vi "AB_RW_Project_Source_ExportedAssemblyVI.vi"(7 "action":T5, 8 "error in (no error)":errorcluster, 9 "index in":i32, 10 "dataSource in":T2, 11 "buildObject":T1) -> (0 "error out":errorcluster, 1 "index out":i32, 2 "dataSource out":T2, 3 "buildObject out":T1)   [LabVIEW 2020]
doc: "Reads and writes the data to the object property bag."
uses:
  <vilib>/AppBuilder/RW_Project/AB_RW_Project_PropBag_Action.ctl
  <vilib>/AppBuilder/RW_Project/AB_RW_Project_Source_ExportedAssemblyVI_Data.ctl
  <vilib>/AppBuilder/AB_InteropAssembly_DistVI_Proto_Info.ctl
  <vilib>/AppBuilder/IOStatus.ctl
  <resource>/Framework/Providers/API/ItemRef.ctl
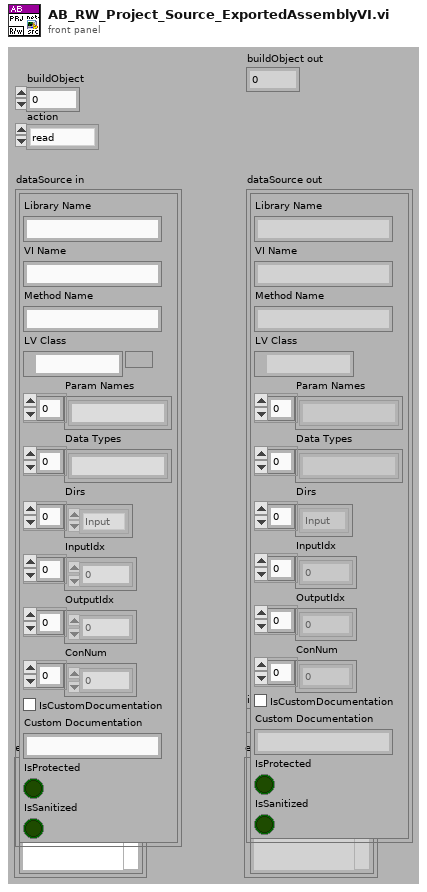
[diagram p1: front panel]
types:
  T1 = typedef "ItemRef.ctl" = u64
  T2 = typedef "AB_RW_Project_Source_ExportedAssemblyVI_Data.ctl" = cluster{"ExportAssemblyVIinfo":T3}
  T3 = typedef "AB_InteropAssembly_DistVI_Proto_Info.ctl" = cluster{"Library Name":string, "VI Name":string, "Method Name":string, "LV Class":path, "Param Names":string[], "Data Types":string[], "Dirs":T4[], "InputIdx":i32[], "OutputIdx":i32[], "ConNum":i8[], "IsCustomDocumentation":bool, "Custom Documentation":string, "IsProtected":bool, "IsSanitized":bool}
  T4 = typedef "IOStatus.ctl" = enum16{"Input", "Output", "Input/Output", "InputDeleted", "OutputDeleted", "IODeleted", "ErrorClusterIn", "ErrorClusterOut"}
  T5 = typedef "AB_RW_Project_PropBag_Action.ctl" = enum16{"read", "write", "clear", "readPrevious", "writePrevious", "clearPrevious"}
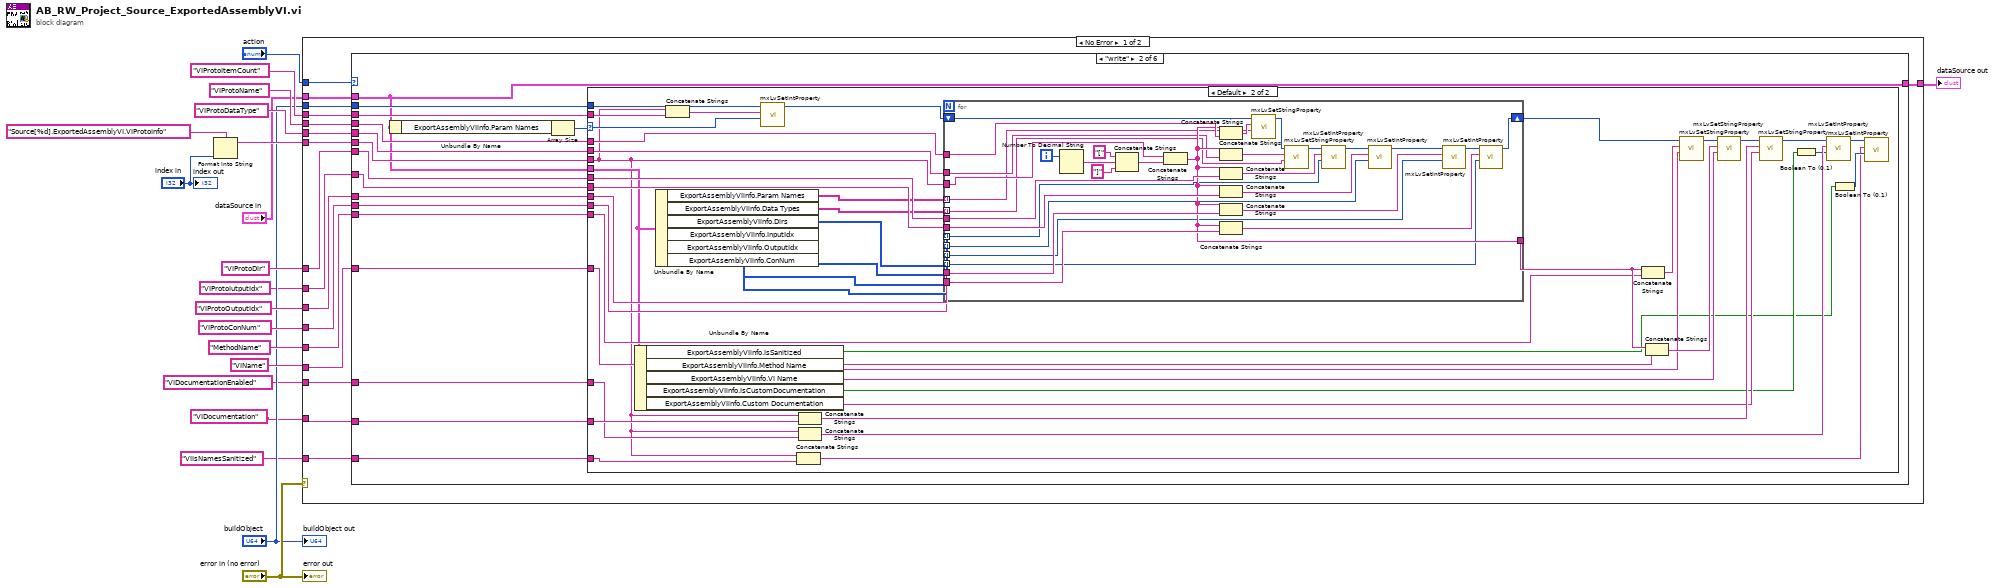
[diagram p0: block diagram]
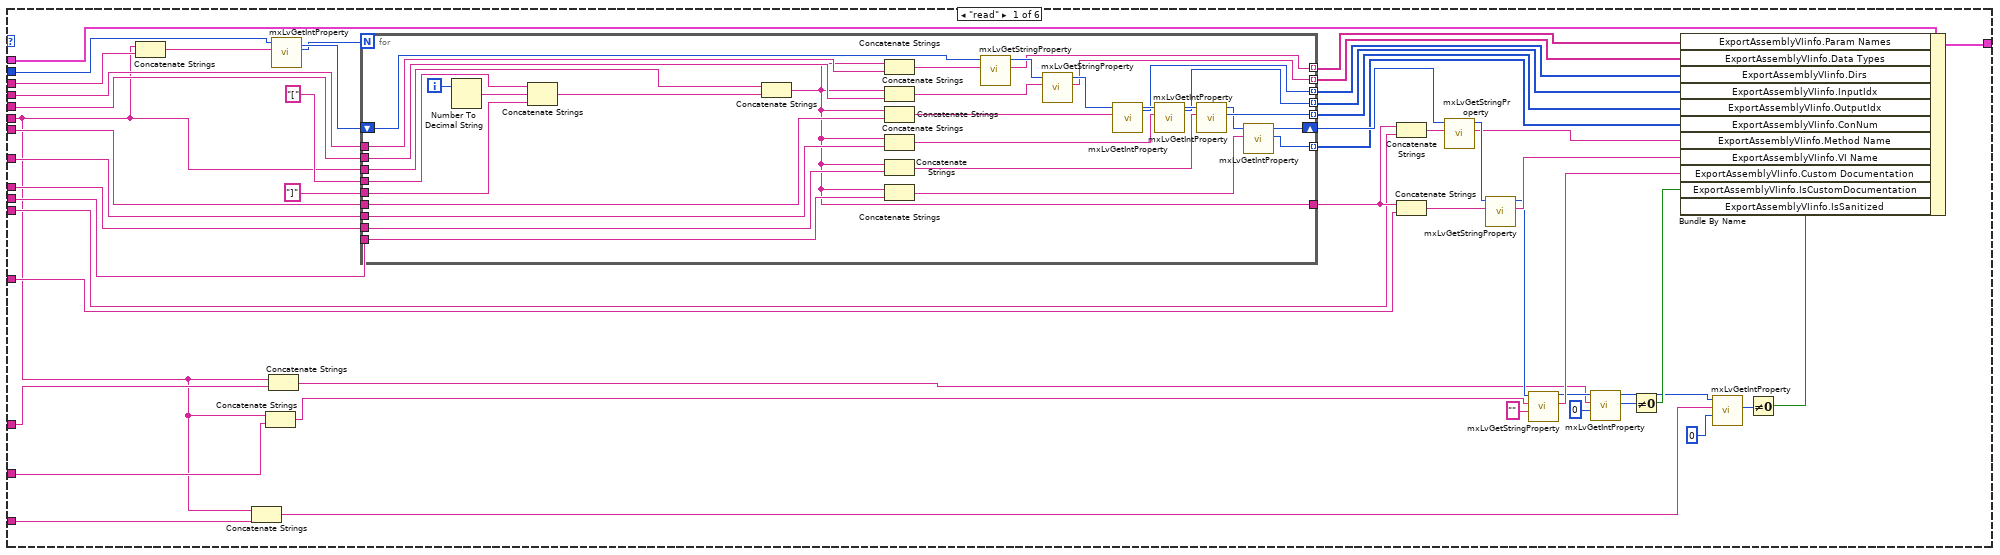
[diagram p2: hidden frame]
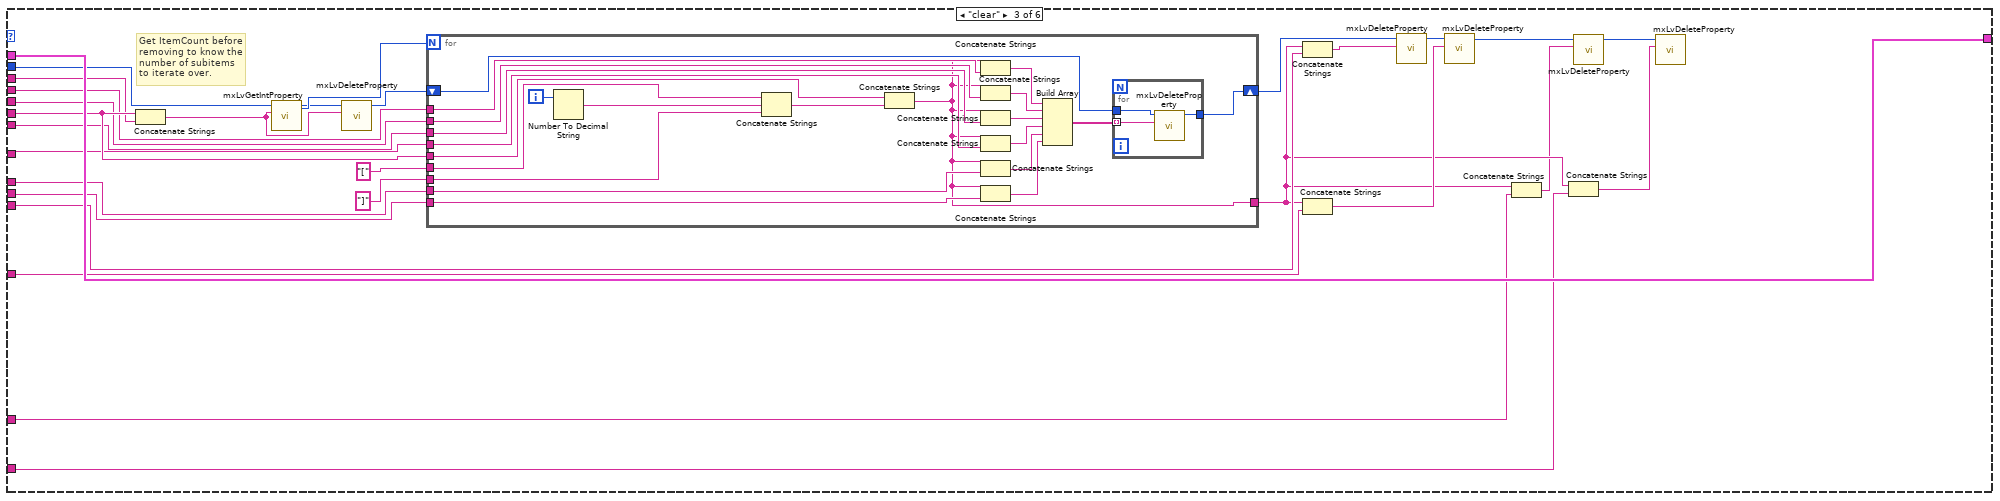
[diagram p4: hidden frame]
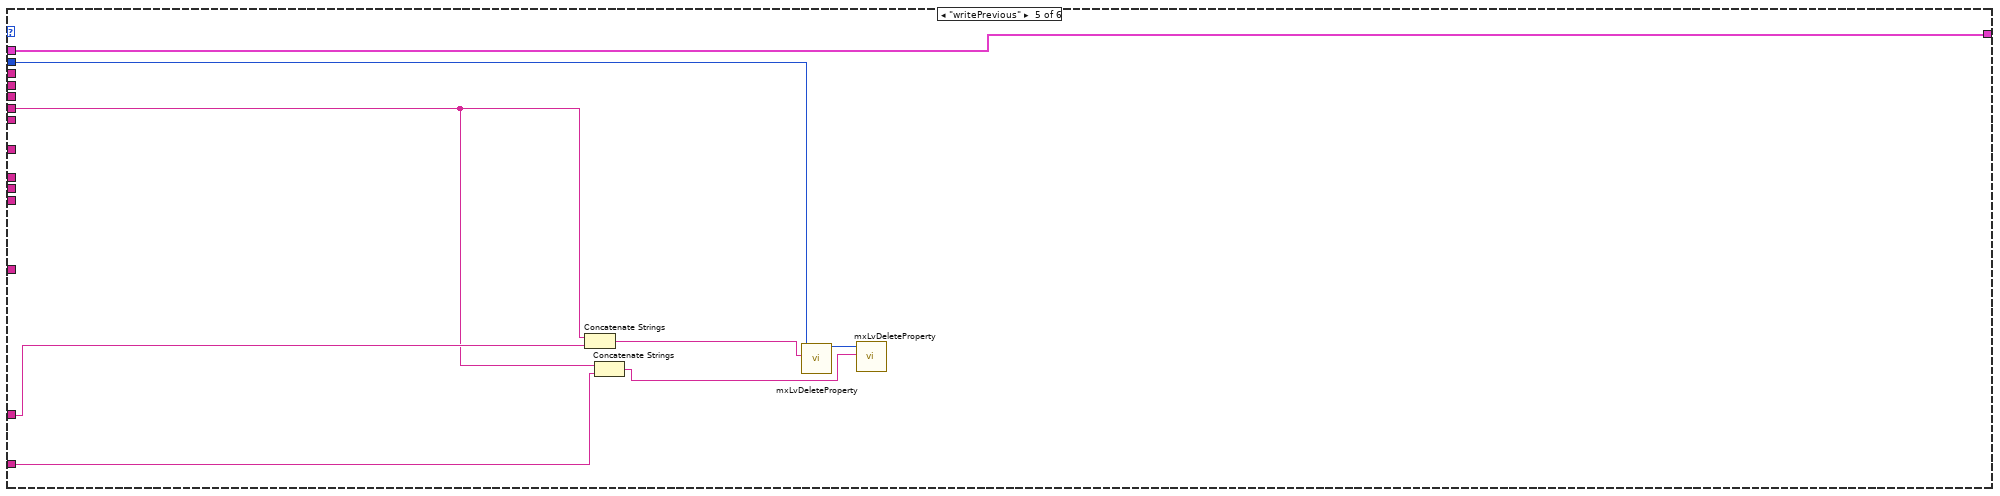
[diagram p6: hidden frame]
diagram:
  n1 = Format Into String(format string="Source[%d].ExportedAssemblyVI.VIProtoInfo", "index in") -> (resulting string=w18:string)  [unwired: 2 in, 1 out]
  n2 = case shown="No Error" "error in (no error)" {
    tunnel: "action" -> [w37 _]
    tunnel: "dataSource in" -> [w36 w273]
    tunnel: w18 -> [w35 _]
    tunnel: "buildObject" -> [w34 _]
    tunnel: [w33 w273] -> w6
    tunnel: "VIProtoItemCount" -> [w32 _]
    tunnel: "VIProtoName" ("string") -> [w31 _]
    tunnel: "VIProtoDataType" ("string") -> [w30 _]
    tunnel: "VIProtoDir" ("string") -> [w29 _]
    tunnel: "VIProtoOutputIdx" ("string") -> [w28 _]
    tunnel: "VIProtoConNum" ("string") -> [w27 _]
    tunnel: "MethodName" -> [w26 _]
    tunnel: "VIName" -> [w25 _]
    tunnel: "VIProtoIutputIdx" ("string") -> [w24 _]
    tunnel: "VIDocumentation" -> [w23 _]
    tunnel: "VIDocumentationEnabled" -> [w22 _]
    tunnel: "VIIsNamesSanitized" -> [w21 _]
    frame No Error {
      n3 = case shown="\"write\"" w37 {
        tunnel: w34 -> [w70 w132 w217 _ w267 _]
        tunnel: w36 -> [w57 w121 w237 w263 w271 w272]
        tunnel: w35 -> [w40 w133 w236 _ w266 _]
        tunnel: [w56 w121 w237 w263 w271 w272] -> w33
        tunnel: w32 -> [w78 w130 w235 _ _ _]
        tunnel: w31 -> [w77 w131 w224 _ _ _]
        tunnel: w30 -> [w76 w128 w223 _ _ _]
        tunnel: w29 -> [w75 w127 w222 _ _ _]
        tunnel: w28 -> [w74 w126 w221 _ _ _]
        tunnel: w27 -> [w73 w125 w220 _ _ _]
        tunnel: w26 -> [w72 w124 w218 _ _ _]
        tunnel: w25 -> [w71 w123 w219 _ _ _]
        tunnel: w24 -> [w69 w122 w216 _ _ _]
        tunnel: w23 -> [w55 w120 w210 _ w265 _]
        tunnel: w22 -> [w54 w119 w211 _ w270 _]
        tunnel: w21 -> [w39 w118 _ _ _ _]
        frame "read" {
          n4 = Concatenate Strings(w40, w78) -> (w84:string)
          n5 = Concatenate Strings(w40, w39) -> (w38:string)
          n6 = Concatenate Strings(w40, w55) -> (w53:string)
          n7 = Concatenate Strings(w40, w54) -> (w47:string)
          n8 = call <resource>:"mxLvGetIntProperty.vi"("Tag"=w84, "Item"=w70) -> ("Value"=w79:i32, "Item"=w83:T1)  [unwired: 1 in, 7 out]
          n9 = for {
            N: w79 -> [_]
            tunnel: "[" -> [w116]
            tunnel: "]" -> [w115]
            tunnel: w40 -> [w111]
            tunnel: [w100] -> w80
            shift-right: [w93] -> w68
            shift-left: w83 -> [w113]
            tunnel: w77 -> [w106]
            tunnel: w76 -> [w105]
            tunnel: w75 -> [w104]
            tunnel: w74 -> [w103]
            tunnel: w73 -> [w102]
            tunnel: w69 -> [w101]
            tunnel: [w92] -> w65 mode=indexing
            tunnel: [w91] -> w64 mode=indexing
            tunnel: [w90] -> w63 mode=indexing
            tunnel: [w89] -> w62 mode=indexing
            tunnel: [w88] -> w61 mode=indexing
            tunnel: [w87] -> w60 mode=indexing
            i -> [w114]
            n10 = Number To Decimal String(number=w114) -> (decimal integer string=w117:string)  [unwired: 1 out]
            n11 = Concatenate Strings(w116, w117, w115) -> (w110:string)
            n12 = Concatenate Strings(w111, w110) -> (w100:string)
            n13 = Concatenate Strings(w100, w106) -> (w112:string)
            n14 = Concatenate Strings(w100, w105) -> (w97:string)
            n15 = Concatenate Strings(w100, w104) -> (w109:string)
            n16 = Concatenate Strings(w100, w101) -> (w94:string)
            n17 = Concatenate Strings(w100, w103) -> (w108:string)
            n18 = Concatenate Strings(w100, w102) -> (w107:string)
            n19 = call <resource>:"mxLvGetStringProperty.vi"("Tag"=w112, "Item"=w113) -> ("Value"=w92:string, "Item"=w99:T1)  [unwired: 1 in, 7 out]
            n20 = call <resource>:"mxLvGetStringProperty.vi"("Tag"=w97, "Item"=w99) -> ("Value"=w91:string, "Item"=w98:T1)  [unwired: 1 in, 7 out]
            n21 = call <resource>:"mxLvGetIntProperty.vi"("Tag"=w109, "Item"=w98) -> ("Value"=w90:i32, "Item"=w95:T1)  [unwired: 1 in, 7 out]
            n22 = call <resource>:"mxLvGetIntProperty.vi"("Tag"=w94, "Item"=w95) -> ("Value"=w89:i32, "Item"=w96:T1)  [unwired: 1 in, 7 out]
            n23 = call <resource>:"mxLvGetIntProperty.vi"("Tag"=w108, "Item"=w96) -> ("Value"=w88:i32, "Item"=w86:T1)  [unwired: 1 in, 7 out]
            n24 = call <resource>:"mxLvGetIntProperty.vi"("Tag"=w107, "Item"=w86) -> ("Value"=w87:i32, "Item"=w93:T1)  [unwired: 1 in, 7 out]
          }
          n25 = Concatenate Strings(w80, w72) -> (w66:string)
          n26 = Concatenate Strings(w80, w71) -> (w85:string)
          n27 = call <resource>:"mxLvGetStringProperty.vi"("Tag"=w66, "Item"=w68) -> ("Value"=w59:string, "Item"=w67:T1)  [unwired: 1 in, 7 out]
          n28 = call <resource>:"mxLvGetStringProperty.vi"("Tag"=w85, "Item"=w67) -> ("Value"=w58:string, "Item"=w51:T1)  [unwired: 1 in, 7 out]
          n29 = call <resource>:"mxLvGetStringProperty.vi"("Default Value (\"\")"="" ("Default Value (\"\")"), "Tag"=w53, "Item"=w51) -> ("Value"=w50:string, "Item"=w49:T1)  [unwired: 1 in, 6 out]
          n30 = call <resource>:"mxLvGetIntProperty.vi"("Default Value (0)"=0, "Tag"=w47, "Item"=w49) -> ("Value"=w46:i32, "Item"=w41:T1)  [unwired: 1 in, 6 out]
          n31 = Not Equal To 0?(x=w46) -> (x != 0?=w45:bool)
          n32 = call <resource>:"mxLvGetIntProperty.vi"("Default Value (0)"=0, "Tag"=w38, "Item"=w41) -> ("Value"=w43:i32)  [unwired: 1 in, 7 out]
          n33 = Not Equal To 0?(x=w43) -> (x != 0?=w42:bool)
          n34 = Bundle By Name(cluster=w57, "ExportAssemblyVIinfo.Param Names"=w65, "ExportAssemblyVIinfo.Data Types"=w64, "ExportAssemblyVIinfo.Dirs"=w63, "ExportAssemblyVIinfo.InputIdx"=w62, "ExportAssemblyVIinfo.OutputIdx"=w61, "ExportAssemblyVIinfo.ConNum"=w60, "ExportAssemblyVIinfo.Method Name"=w59, "ExportAssemblyVIinfo.VI Name"=w58, "ExportAssemblyVIinfo.Custom Documentation"=w50, "ExportAssemblyVIinfo.IsCustomDocumentation"=w45, "ExportAssemblyVIinfo.IsSanitized"=w42) -> (w56:T2)
        }
        frame "write" {
          n35 = Unbundle By Name(w121) -> ("ExportAssemblyVIinfo.Param Names"=w134:string[])
          n36 = Array Size(array=w134) -> (size(s)=w129:i32)
          n37 = case shown="Default" w129 {
            selector: w129 -> [_ w171]
            tunnel: w132 -> [_ w168]
            tunnel: w133 -> [_ w139]
            tunnel: w131 -> [_ w173]
            tunnel: w130 -> [_ w172]
            tunnel: w128 -> [_ w167]
            tunnel: w127 -> [_ w166]
            tunnel: w126 -> [_ w164]
            tunnel: w125 -> [_ w163]
            tunnel: w124 -> [_ w170]
            tunnel: w123 -> [_ w169]
            tunnel: w122 -> [_ w165]
            tunnel: w121 -> [_ w147]
            tunnel: w120 -> [_ w159]
            tunnel: w119 -> [_ w158]
            tunnel: w118 -> [_ w140]
            frame 0 {
              # "If default, then don't write anything out."
            }
            frame Default {
              n38 = Unbundle By Name(w147) -> ("ExportAssemblyVIinfo.IsSanitized"=w136:bool, "ExportAssemblyVIinfo.Method Name"=w143:string, "ExportAssemblyVIinfo.VI Name"=w142:string, "ExportAssemblyVIinfo.IsCustomDocumentation"=w141:bool, "ExportAssemblyVIinfo.Custom Documentation"=w146:string)
              n39 = Unbundle By Name(w147) -> ("ExportAssemblyVIinfo.Param Names"=w145:string[], "ExportAssemblyVIinfo.Data Types"=w144:string[], "ExportAssemblyVIinfo.Dirs"=w151:T4[], "ExportAssemblyVIinfo.InputIdx"=w150:i32[], "ExportAssemblyVIinfo.OutputIdx"=w149:i32[], "ExportAssemblyVIinfo.ConNum"=w148:i8[])
              n40 = Concatenate Strings(w139, w172) -> (w175:string)
              n41 = call <resource>:"mxLvSetIntProperty.vi"("Value (0)"=w171, "Tag"=w175, "Item"=w168) -> ("Item"=w156:T1)  [unwired: 2 in, 6 out]
              n42 = Concatenate Strings(w139, w140) -> (w135:string)
              n43 = Concatenate Strings(w139, w159) -> (w157:string)
              n44 = Concatenate Strings(w139, w158) -> (w155:string)
              n45 = for {
                tunnel: w139 -> [w204]
                tunnel: [w191] -> w174
                shift-right: [w197] -> w162
                shift-left: w156 -> [w206]
                tunnel: w173 -> [w196]
                tunnel: w166 -> [w195]
                tunnel: w165 -> [w194]
                tunnel: w164 -> [w193]
                tunnel: w163 -> [w192]
                tunnel: w167 -> [w190]
                tunnel: w145 -> [w186] mode=indexing
                tunnel: w144 -> [w185] mode=indexing
                tunnel: w151 -> [w184] mode=indexing
                tunnel: w150 -> [w183] mode=indexing
                tunnel: w149 -> [w181] mode=indexing
                tunnel: w148 -> [w180] mode=indexing
                i -> [w207]
                n46 = Number To Decimal String(number=w207) -> (decimal integer string=w208:string)  [unwired: 1 out]
                n47 = Concatenate Strings("[", w208, "]") -> (w203:string)
                n48 = Concatenate Strings(w204, w203) -> (w191:string)
                n49 = Concatenate Strings(w191, w196) -> (w205:string)
                n50 = Concatenate Strings(w191, w190) -> (w187:string)
                n51 = Concatenate Strings(w191, w195) -> (w202:string)
                n52 = Concatenate Strings(w191, w194) -> (w182:string)
                n53 = Concatenate Strings(w191, w193) -> (w199:string)
                n54 = Concatenate Strings(w191, w192) -> (w198:string)
                n55 = call <resource>:"mxLvSetStringProperty.vi"("Value (\"\")"=w186, "Tag"=w205, "Item"=w206) -> ("Item"=w189:T1)  [unwired: 2 in, 6 out]
                n56 = call <resource>:"mxLvSetStringProperty.vi"("Value (\"\")"=w185, "Tag"=w187, "Item"=w189) -> ("Item"=w188:T1)  [unwired: 2 in, 6 out]
                n57 = call <resource>:"mxLvSetIntProperty.vi"("Value (0)"=w184, "Tag"=w202, "Item"=w188) -> ("Item"=w201:T1)  [unwired: 2 in, 6 out]
                n58 = call <resource>:"mxLvSetIntProperty.vi"("Value (0)"=w183, "Tag"=w182, "Item"=w201) -> ("Item"=w200:T1)  [unwired: 2 in, 6 out]
                n59 = call <resource>:"mxLvSetIntProperty.vi"("Value (0)"=w181, "Tag"=w199, "Item"=w200) -> ("Item"=w179:T1)  [unwired: 2 in, 6 out]
                n60 = call <resource>:"mxLvSetIntProperty.vi"("Value (0)"=w180, "Tag"=w198, "Item"=w179) -> ("Item"=w197:T1)  [unwired: 2 in, 6 out]
              }
              n61 = Concatenate Strings(w174, w170) -> (w160:string)
              n62 = Concatenate Strings(w174, w169) -> (w176:string)
              n63 = call <resource>:"mxLvSetStringProperty.vi"("Value (\"\")"=w143, "Tag"=w160, "Item"=w162) -> ("Item"=w161:T1)  [unwired: 2 in, 6 out]
              n64 = call <resource>:"mxLvSetStringProperty.vi"("Value (\"\")"=w142, "Tag"=w176, "Item"=w161) -> ("Item"=w152:T1)  [unwired: 2 in, 6 out]
              n65 = call <resource>:"mxLvSetStringProperty.vi"("Value (\"\")"=w146, "Tag"=w157, "Item"=w152) -> ("Item"=w154:T1)  [unwired: 2 in, 6 out]
              n66 = Boolean To (0,1)(Boolean=w141) -> (0, 1=w153:i16)
              n67 = call <resource>:"mxLvSetIntProperty.vi"("Value (0)"=w153, "Tag"=w155, "Item"=w154) -> ("Item"=w137:T1)  [unwired: 2 in, 6 out]
              n68 = Boolean To (0,1)(Boolean=w136) -> (0, 1=w138:i16)
              n69 = call <resource>:"mxLvSetIntProperty.vi"("Value (0)"=w138, "Tag"=w135, "Item"=w137) -> ()  [unwired: 2 in, 7 out]
            }
          }
        }
        frame "clear" {
          # "Get ItemCount before removing to know the number of subitems to iterate over."
          n70 = Concatenate Strings(w236, w235) -> (w225:string)
          n71 = call <resource>:"mxLvGetIntProperty.vi"("Tag"=w225, "Item"=w217) -> ("Value"=w227:i32, "Item"=w226:T1)  [unwired: 1 in, 7 out]
          n72 = call <resource>:"mxLvDeleteProperty.vi"("Tag"=w225, "Item"=w226) -> ("Item"=w232:T1)  [unwired: 2 in, 7 out]
          n73 = for {
            N: w227 -> [_]
            tunnel: "[" -> [w258]
            tunnel: "]" -> [w257]
            tunnel: w236 -> [w255]
            tunnel: [w247] -> w214
            shift-right: [w238] -> w229
            shift-left: w232 -> [w240]
            tunnel: w224 -> [w253]
            tunnel: w223 -> [w252]
            tunnel: w222 -> [w251]
            tunnel: w221 -> [w250]
            tunnel: w220 -> [w249]
            tunnel: w216 -> [w248]
            i -> [w256]
            n74 = Number To Decimal String(number=w256) -> (decimal integer string=w259:string)  [unwired: 1 out]
            n75 = Concatenate Strings(w258, w259, w257) -> (w254:string)
            n76 = Concatenate Strings(w255, w254) -> (w247:string)
            n77 = Concatenate Strings(w247, w253) -> (w246:string)
            n78 = Concatenate Strings(w247, w252) -> (w245:string)
            n79 = Concatenate Strings(w247, w251) -> (w244:string)
            n80 = Concatenate Strings(w247, w248) -> (w243:string)
            n81 = Concatenate Strings(w247, w250) -> (w242:string)
            n82 = Concatenate Strings(w247, w249) -> (w241:string)
            n83 = Build Array(w246, w245, w244, w243, w242, w241) -> (w239:string[])
            n84 = for {
              tunnel: w240 -> [w262]
              tunnel: w239 -> [w261] mode=indexing
              tunnel: [w260] -> w238
              n85 = call <resource>:"mxLvDeleteProperty.vi"("Tag"=w261, "Item"=w262) -> ("Item"=w260:T1)  [unwired: 2 in, 7 out]
            }
          }
          n86 = Concatenate Strings(w214, w218) -> (w233:string)
          n87 = Concatenate Strings(w214, w219) -> (w234:string)
          n88 = call <resource>:"mxLvDeleteProperty.vi"("Tag"=w233, "Item"=w229) -> ("Item"=w228:T1)  [unwired: 2 in, 7 out]
          n89 = call <resource>:"mxLvDeleteProperty.vi"("Tag"=w234, "Item"=w228) -> ("Item"=w209:T1)  [unwired: 2 in, 7 out]
          n90 = Concatenate Strings(w214, w211) -> (w212:string)
          n91 = Concatenate Strings(w214, w210) -> (w213:string)
          n92 = call <resource>:"mxLvDeleteProperty.vi"("Tag"=w212, "Item"=w209) -> ("Item"=w215:T1)  [unwired: 2 in, 7 out]
          n93 = call <resource>:"mxLvDeleteProperty.vi"("Tag"=w213, "Item"=w215) -> ()  [unwired: 2 in, 8 out]
        }
        frame "readPrevious" {
        }
        frame "writePrevious" {
          n94 = Concatenate Strings(w266, w270) -> (w269:string)
          n95 = Concatenate Strings(w266, w265) -> (w264:string)
          n96 = call <resource>:"mxLvDeleteProperty.vi"("Tag"=w269, "Item"=w267) -> ("Item"=w268:T1)  [unwired: 2 in, 7 out]
          n97 = call <resource>:"mxLvDeleteProperty.vi"("Tag"=w264, "Item"=w268) -> ()  [unwired: 2 in, 8 out]
        }
        frame "clearPrevious" {
        }
      }
    }
    frame Error {
    }
  }
  "dataSource out" <- w6
  "error out" <- "error in (no error)"
  "index out" <- "index in"
  "buildObject out" <- "buildObject"
